vi "Move Cost.vi"(8 "Room Slot in":i32, 9 "Destination Position in":i32, 10 "Source Position in":i32, 11 "Amphipod Type Index in":i32) -> (0 "Room Slot out":i32, 1 "Destination Position out":i32, 2 "Source Position out":i32, 3 "Amphipod Type Index out":i32, 4 "Move Cost":u64)   [LabVIEW 2019, in "23.lvlib" / "State.lvclass"]
uses:
  State.lvclass
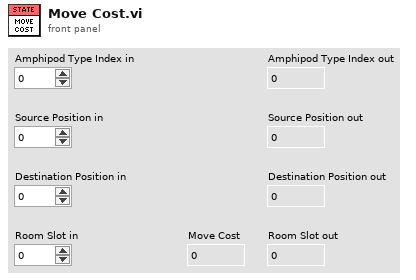
[diagram p1: front panel]
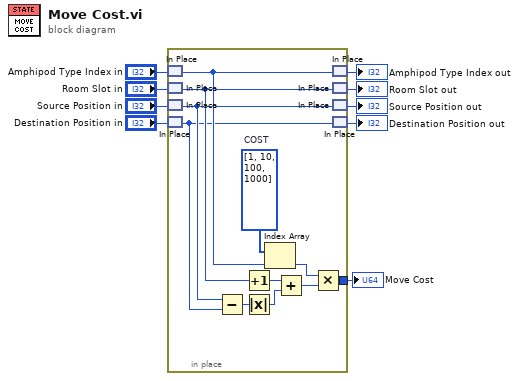
[diagram p0: block diagram]
diagram:
  n1 = in-place {
    in-place-border: [w19] -> w9
    w20 = u64[] [1, 10, 100, 1000]  # COST
    n2 = in-place-match #1("Amphipod Type Index in") -> (w13:i32)
    n3 = in-place-match #2("Room Slot in") -> (w12:i32)
    n4 = in-place-match #3("Source Position in") -> (w11:i32)
    n5 = in-place-match #4("Destination Position in") -> (w10:i32)
    n6 = Subtract(x=w11, y=w10) -> (x-y=w14:i32)
    n7 = Increment(x=w12) -> (x+1=w16:i32)
    n8 = Absolute Value(x=w14) -> (abs(x)=w15:i32)
    n9 = Index Array(array=w20, index=w13) -> (element=w18:u64)
    n10 = Add(x=w16, y=w15) -> (x+y=w17:i32)
    n11 = Multiply(x=w18, y=w17) -> (x*y=w19:u64)
    n12 = in-place-match #1(w13) -> (→"Amphipod Type Index out":i32)
    n13 = in-place-match #2(w12) -> (→"Room Slot out":i32)
    n14 = in-place-match #3(w11) -> (→"Source Position out":i32)
    n15 = in-place-match #4(w10) -> (→"Destination Position out":i32)
  }
  "Move Cost" <- w9
